vi "convertor imagine2.vi"() -> ()   [LabVIEW 2024]
uses:
  <vilib>/vision/NI_Vision_Development_Module.lvlib
  <vilib>/MakerHub/Toolbox/LMH-Toolbox.lvlib
panel:
  out "substring 3":string
  out "substring":string
  out "filenames":string[](array[string])
  out "\\Proiect RN":path
  out "Image 2":T1(plugin-control)
  out "path citire":path
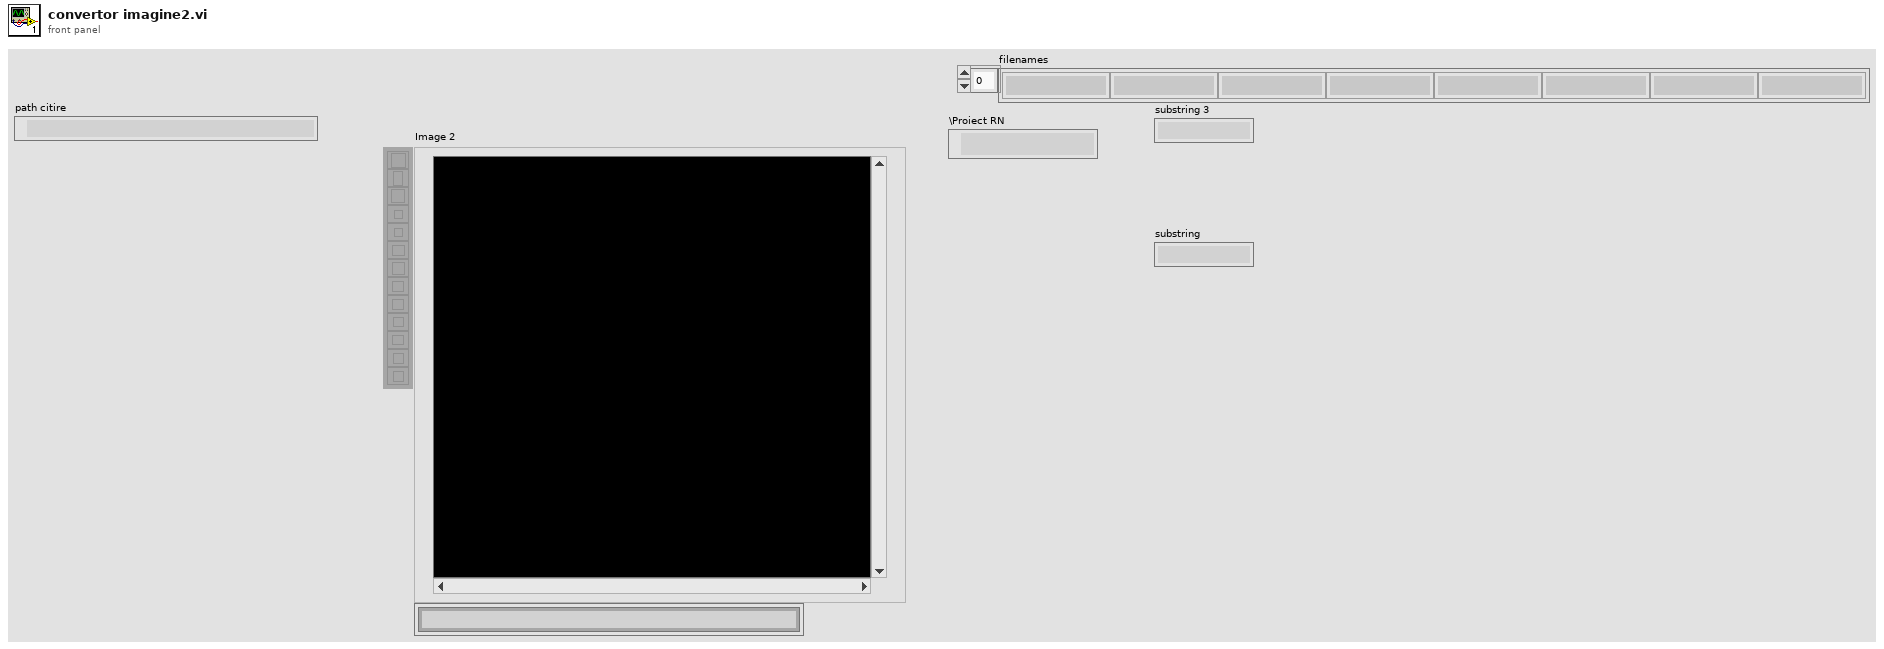
[diagram p1: front panel]
types:
  T1 = typedef "IMAQ Image.ctl" = refnum<image>
  T2 = typedef "Color (U64)" = cluster{"Plane 3 (Blue)":u16, "Plane 2 (Green)":u16, "Plane 1 (Red)":u16, "Plane 4 (alpha)":u16}
  T3 = typedef "Image Type" = u32
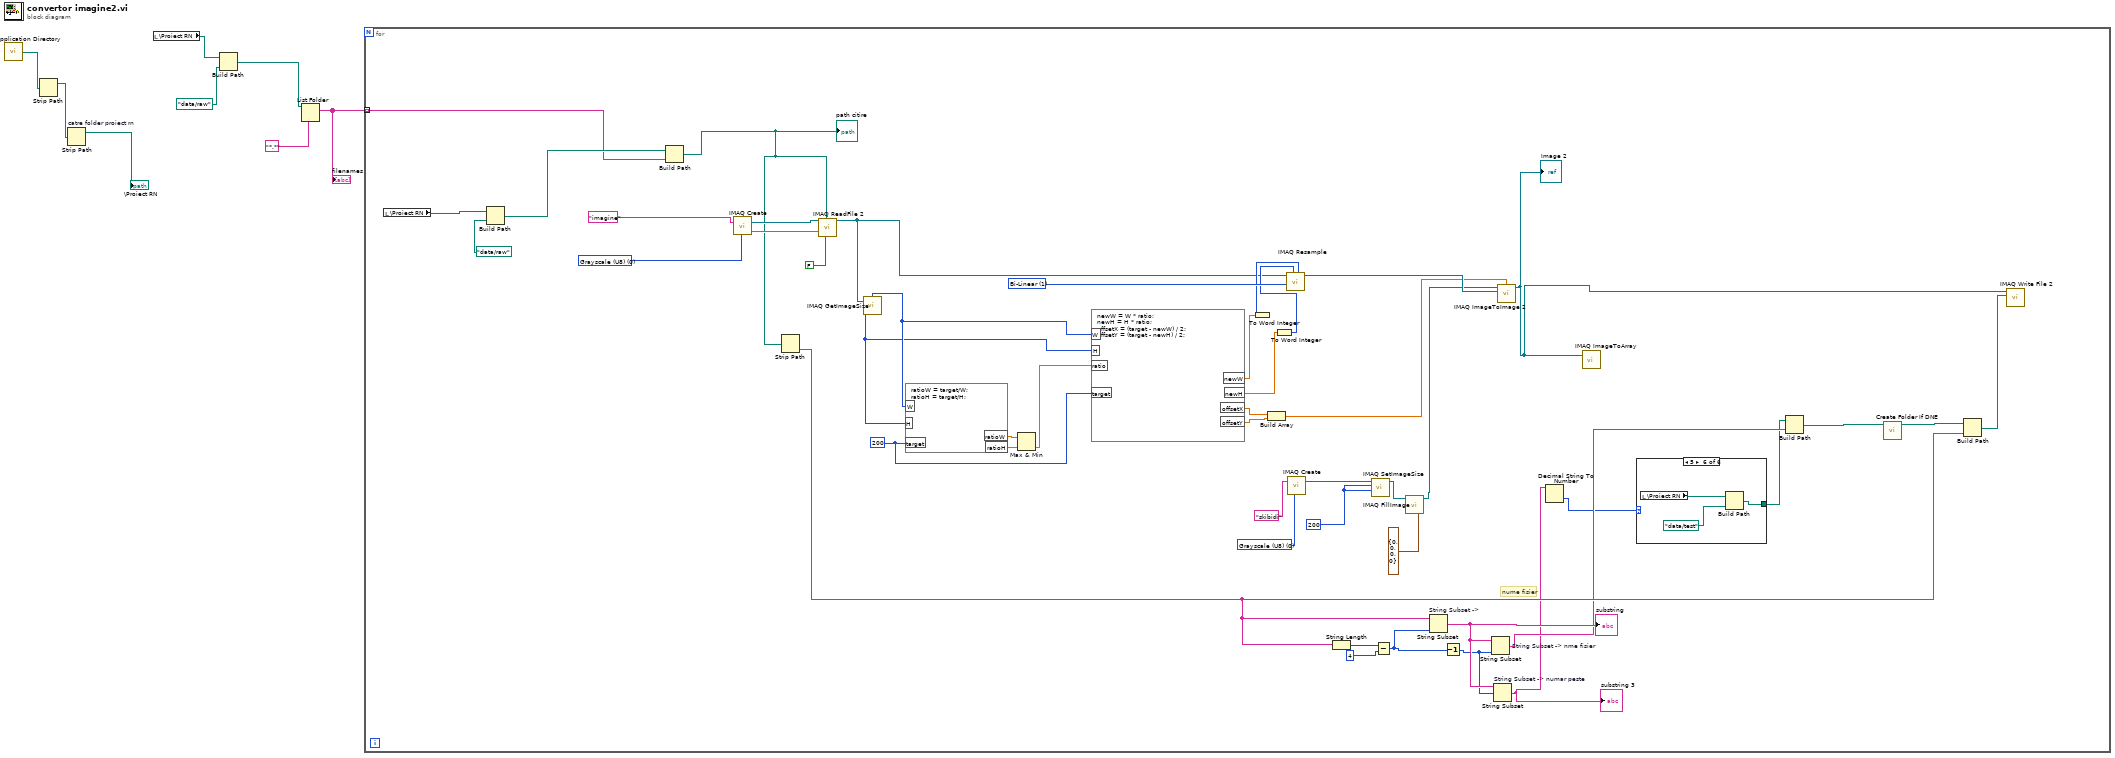
[diagram p0: block diagram]
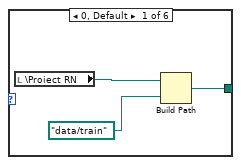
[diagram p2: hidden frame]
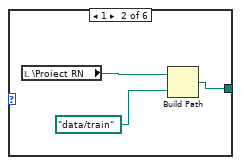
[diagram p3: hidden frame]
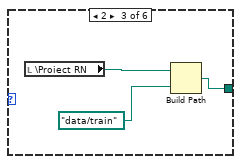
[diagram p4: hidden frame]
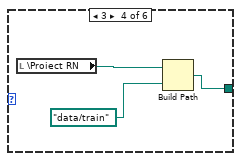
[diagram p5: hidden frame]
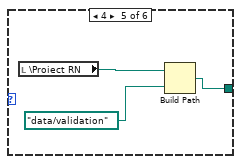
[diagram p6: hidden frame]
diagram:
  n1 = call <vilib>:"Application Directory.vi"() -> ("Application Directory"=w7:path)
  n2 = Strip Path(path=w7) -> (stripped path=w8:path)  [unwired: 1 out]
  n3 = Strip Path "catre folder proiect rn"(path=w8) -> (stripped path=→"\\Proiect RN":path)  [unwired: 1 out]
  n4 = local read "\\Proiect RN"() -> (w4:path)
  n5 = Build Path(base path=w4, name or relative path=path "data/raw") -> (appended path=w3:path)
  n6 = List Folder(path=w3, pattern="*.*") -> (filenames=w1:string[])  [unwired: 2 in, 3 out]
  "filenames" <- w1
  n7 = for {
    tunnel: w1 -> [w21] mode=indexing
    w37 = 200 ("Y Resolution")
    w39 = T3 0 items=["Grayscale (U8)", "Grayscale (I16)", "Grayscale (SGL)", "Complex (CSG)", "RGB (U32)", "HSL (U32)", "RGB (U64)", "Grayscale (U16)"] ("Image Type")
    w44 = u32 1 items=["Zero Order", "Bi-Linear", "Quadratic", "Cubic Spline"] ("Interpolation Type")
    w45 = 200
    w54 = T3 0 items=["Grayscale (U8)", "Grayscale (I16)", "Grayscale (SGL)", "Complex (CSG)", "RGB (U32)", "HSL (U32)", "RGB (U64)", "Grayscale (U16)"] ("Image Type")
    # "nume fisier"
    n8 = local read "\\Proiect RN"() -> (w25:path)
    n9 = Build Path(base path=w25, name or relative path=path "data/raw") -> (appended path=w23:path)
    n10 = Build Path(base path=w23, name or relative path=w21) -> (appended path=w22:path)
    "path citire" <- w22
    n11 = call "IMAQ Create"("Image Name"="imagine", "Image Type"=w54) -> ("New Image"=w51:T1, "error out"=w53:errorcluster)  [unwired: 3 in]
    n12 = Strip Path(path=w22) -> (name=w18:string)  [unwired: 1 out]
    n13 = call "IMAQ ReadFile 2"("Use File Path Image Type"=FALSE, "File Path"=w22, "error in (no error)"=w53, "Image"=w51) -> ("Image Out"=w29:T1)  [unwired: 3 in, 4 out]
    n14 = call "IMAQ GetImageSize"("Image"=w29) -> ("Y Resolution"=w46:i32, "X Resolution"=w47:i32)  [unwired: 3 in, 1 out]
    n15 = formula code="ratioW = target/W;\nratioH = target/H;"("W"=w47, "H"=w46, "target"=w45) -> ("ratioW"=w50:dbl, "ratioH"=w49:dbl)
    n16 = Max & Min(x=w50, y=w49) -> (min(x,y)=w48:dbl)  [unwired: 1 out]
    n17 = formula code="newW = W * ratio;\nnewH = H * ratio;\noffsetX = (target - newW) / 2;\noffsetY = (target - newH) / 2;"("ratio"=w48, "W"=w47, "H"=w46, "target"=w45) -> ("newW"=w41:dbl, "newH"=w43:dbl, "offsetX"=w30:dbl, "offsetY"=w31:dbl)
    n18 = To Word Integer(number=w41) -> (16bit integer=w40:i16)
    n19 = Build Array(w30, w31) -> (w28:dbl[])
    n20 = To Word Integer(number=w43) -> (16bit integer=w42:i16)
    n21 = call "IMAQ Resample"("X Resolution"=w40, "Y Resolution"=w42, "Interpolation Type"=w44, "Image Src"=w29) -> ("Image Dst Out"=w35:T1)  [unwired: 6 in, 1 out]
    n22 = call "IMAQ Create"("Image Name"="skibidi", "Image Type"=w39) -> ("New Image"=w38:T1)  [unwired: 3 in, 1 out]
    n23 = String Length(string=w18) -> (length=w20:i32)
    n24 = call "IMAQ SetImageSize"("Y Resolution"=w37, "X Resolution"=w37, "Image"=w38) -> ("Image Out"=w33:T1)  [unwired: 2 in, 1 out]
    n25 = Subtract(x=w20, y=4) -> (x-y=w16:i32)
    n26 = call "IMAQ FillImage"("Color (U64)"=T2 {"Plane 3 (Blue)"=0, "Plane 2 (Green)"=0, "Plane 1 (Red)"=0, "Plane 4 (alpha)"=0}, "Image"=w33) -> ("Image Out"=w32:T1)  [unwired: 8 in, 1 out]
    n27 = String Subset "String Subset ->"(string=w18, length (rest)=w16) -> (substring=w17:string)  [unwired: 1 in]
    "substring" <- w17
    n28 = Decrement(x=w16) -> (x-1=w15:i32)
    n29 = String Subset "String Subset -> nme fisier"(string=w17, length (rest)=w15) -> (substring=w14:string)  [unwired: 1 in]
    n30 = String Subset "String Subset -> numar peste"(string=w17, offset (0)=w15) -> (substring=w11:string)  [unwired: 1 in]
    "substring 3" <- w11
    n31 = call "IMAQ ImageToImage 2"("Offset Left/Top"=w28, "Image Src (Small)"=w35, "Image Src (Large)"=w32) -> ("Image Dst Out"=w27:T1)  [unwired: 7 in, 1 out]
    "Image 2" <- w27
    n32 = Decimal String To Number(string=w11) -> (number=w10:i32)  [unwired: 2 in, 1 out]
    n33 = call "IMAQ ImageToArray"("Image"=w27) -> ()  [unwired: 3 in, 5 out]
    n34 = case shown="5" w10 {
      tunnel: [w56 w59 w62 w65 w68 w71] -> w9
      frame 0, Default {
        n35 = local read "\\Proiect RN"() -> (w58:path)
        n36 = Build Path(base path=w58, name or relative path=path "data/train") -> (appended path=w56:path)
      }
      frame 1 {
        n37 = local read "\\Proiect RN"() -> (w60:path)
        n38 = Build Path(base path=w60, name or relative path=path "data/train") -> (appended path=w59:path)
      }
      frame 2 {
        n39 = local read "\\Proiect RN"() -> (w63:path)
        n40 = Build Path(base path=w63, name or relative path=path "data/train") -> (appended path=w62:path)
      }
      frame 3 {
        n41 = local read "\\Proiect RN"() -> (w66:path)
        n42 = Build Path(base path=w66, name or relative path=path "data/train") -> (appended path=w65:path)
      }
      frame 4 {
        n43 = local read "\\Proiect RN"() -> (w69:path)
        n44 = Build Path(base path=w69, name or relative path=path "data/validation") -> (appended path=w68:path)
      }
      frame 5 {
        n45 = local read "\\Proiect RN"() -> (w72:path)
        n46 = Build Path(base path=w72, name or relative path=path "data/test") -> (appended path=w71:path)
      }
    }
    n47 = Build Path(base path=w9, name or relative path=w14) -> (appended path=w13:path)
    n48 = call <vilib>:"Create Folder If DNE.vi"("Folder Path"=w13) -> ("Dup Path"=w12:path)  [unwired: 9 in, 1 out]
    n49 = Build Path(base path=w12, name or relative path=w18) -> (appended path=w24:path)
    n50 = call-poly "IMAQ Write File 2"("File Path"=w24, "Image"=w27) -> ()  [unwired: 8 in, 2 out]
  }
